vi "FID Allgemeindaten.vi"(6 "Aktion":T2, 8 "error in (no error)":errorcluster caption="Fehler (Eingang, kein Fehler)", 10 "Switching time":sgl caption="sec" min=0 format="%#.0f", 11 "Mode":T1) -> (0 "error out":errorcluster caption="Fehler (Ausgang)", 3 "FID Allgemein":cluster{"Mode":T1, "Switching time":sgl})   [LabVIEW 2020, in "ABB-EL3000.lvlib" / "FID.lvlib" / "FID Kalibrierung.lvlib"]
uses:
  FID Kalibrierung.lvlib
  Aktion FID Allgemeindaten.ctl
  Modus.ctl
  Allgemein/allgemeine Sub-VIs.lvlib
  FID.lvlib
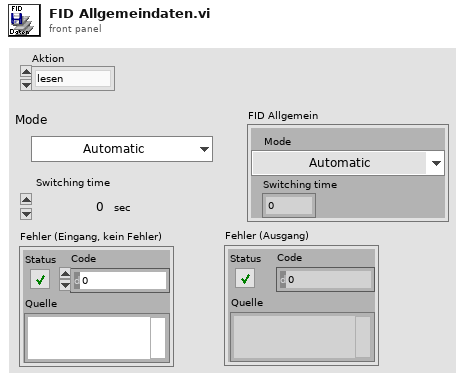
[diagram p1: front panel]
types:
  T1 = typedef "ABB-EL3000.lvlib/FID.lvlib/Modus.ctl" = enum16{"Automatic", "CH4", "THC", "Efficienty measure", "Switching time"}
  T2 = typedef "ABB-EL3000.lvlib/FID.lvlib/FID Kalibrierung.lvlib/Aktion FID Allgemeindaten.ctl" = enum16{"lesen", "Mod", "Time", "laden", "speichern"}
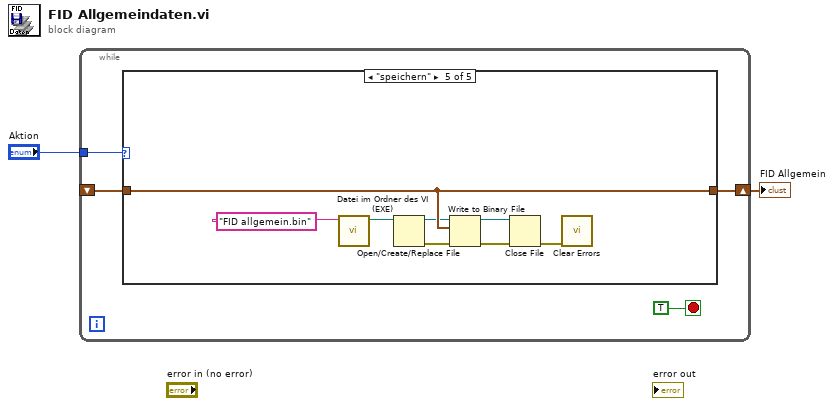
[diagram p0: block diagram]
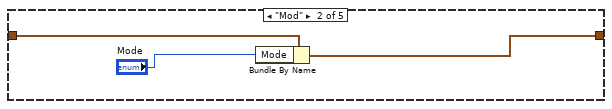
[diagram p3: hidden frame]
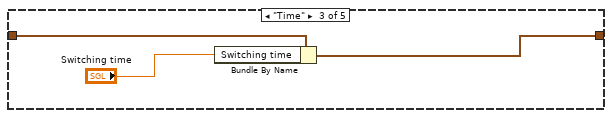
[diagram p4: hidden frame]
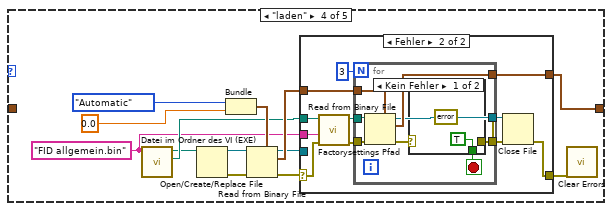
[diagram p5: hidden frame]
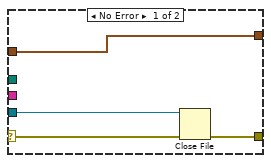
[diagram p6: hidden frame]
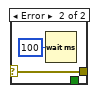
[diagram p7: hidden frame]
diagram:
  n1 = while {
    tunnel: "Aktion" -> [w5]
    shift-right: [w4] -> w1
    shift-left: _ -> [w3]
    stop <- TRUE stop-if-true
    n2 = case shown="\"speichern\"" w5 {
      tunnel: [w7 w8 w12 w17 w61] -> w4
      tunnel: w3 -> [w7 w10 w13 _ w61]
      frame "lesen", Default {
      }
      frame "Mod" {
        n3 = Bundle By Name(cluster=w10, "Mode"="Mode") -> (w8:cluster{"Mode":T1, "Switching time":sgl})
      }
      frame "Time" {
        n4 = Bundle By Name(cluster=w13, "Switching time"="Switching time") -> (w12:cluster{"Mode":T1, "Switching time":sgl})
      }
      frame "laden" {
        w20 = "FID allgemein.bin" ("Dateiname")
        n5 = call "Datei im Ordner des VI (EXE).vi"("Dateiname"=w20) -> ("Ordner des Haupt-VIs"=w21:path, "Dateipfad im Ordner des Haupt-VIs"=w15:path)  [unwired: 8 in, 1 out]
        n6 = Open/Create/Replace File(file path (use dialog)=w15) -> (refnum out=w14:refnum<file>, error out=w16:errorcluster)  [unwired: 5 in, 1 out]
        n7 = Bundle("Mode"=Modus."Automatic", "Switching time"=sgl 0.0) -> (w24:cluster{"Mode":T1, "Switching time":sgl})  [unwired: 1 in]
        n8 = Read from Binary File(5:w24, 8:w16, 11:w14) -> (0:w23:errorcluster, 2:w22:cluster{"Mode":T1, "Switching time":sgl}, 3:w19:refnum<file>)  [unwired: 4 out]
        n9 = case shown="Fehler" w23 {
          selector: w23 -> [w29 w33]
          tunnel: w21 -> [_ w34]
          tunnel: w22 -> [w30 w32]
          tunnel: [w30 w40] -> w17
          tunnel: [w27 w38] -> w18
          tunnel: w19 -> [w28 _]
          tunnel: w20 -> [_ w31]
          frame No Error {
            n10 = Close File(refnum=w28, error in=w29) -> (error out=w27:errorcluster)  [unwired: 1 out]
          }
          frame Error {
            n11 = call "Factorysettings Pfad.vi"("error in (no error)"=w33, "Dateiname"=w31, "Ordner des Haupt-VIs"=w34) -> ("error out"=w35:errorcluster, "Pfad Factorysettings"=w36:path)  [unwired: 7 in]
            n12 = for {
              N: 3 -> [_]
              tunnel: w35 -> [w47]
              tunnel: w36 -> [w46]
              tunnel: [w45] -> w40
              tunnel: [w44] -> w39
              tunnel: [w43] -> w37
              tunnel: w32 -> [w42]
              stop <- w48 stop-if-true
              n13 = Read from Binary File(5:w42, 8:w47, 11:w46) -> (0:w49:errorcluster, 2:w45:cluster{"Mode":T1, "Switching time":sgl}, 3:w43:refnum<file>)  [unwired: 3 in, 1 out]
              n14 = case shown="Kein Fehler" w49 {
                selector: w49 -> [_ w52]
                tunnel: [TRUE _] -> w48
                tunnel: [errorcluster {"status"=FALSE, "code"=0, "source"=""} ("error IO") w52] -> w44
                frame No Error {
                }
                frame Error {
                  n15 = Wait (ms)(milliseconds to wait=u32 100 ("Zu wartende ms")) -> ()  [unwired: 1 out]
                }
              }
            }
            n16 = Close File(refnum=w37, error in=w39) -> (error out=w38:errorcluster)  [unwired: 1 out]
          }
        }
        n17 = call <vilib>:"Clear Errors.vi"("error in (no error)"=w18) -> ()  [unwired: 5 in, 2 out]
      }
      frame "speichern" {
        n18 = call "Datei im Ordner des VI (EXE).vi"("Dateiname"="FID allgemein.bin") -> ("Dateipfad im Ordner des Haupt-VIs"=w59:path)  [unwired: 8 in, 2 out]
        n19 = Open/Create/Replace File(file path (use dialog)=w59) -> (refnum out=w57:refnum<file>, error out=w58:errorcluster)  [unwired: 5 in, 1 out]
        n20 = Write to Binary File(file (use dialog)=w57, data=w61, error in=w58) -> (refnum out=w55:refnum<file>, error out=w56:errorcluster)  [unwired: 4 out]
        n21 = Close File(refnum=w55, error in=w56) -> (error out=w54:errorcluster)  [unwired: 1 out]
        n22 = call <vilib>:"Clear Errors.vi"("error in (no error)"=w54) -> ()  [unwired: 5 in, 2 out]
      }
    }
  }
  "FID Allgemein" <- w1
